vi "Test VI.vi"(9 "y":dbl, 10 "x":dbl) -> (0 "Application:Version Year":string, 1 "Application:Version Number":string, 2 "Application:Name":string, 3 "x+y":dbl)   [LabVIEW 2019]
uses:
  2018.lvlibp
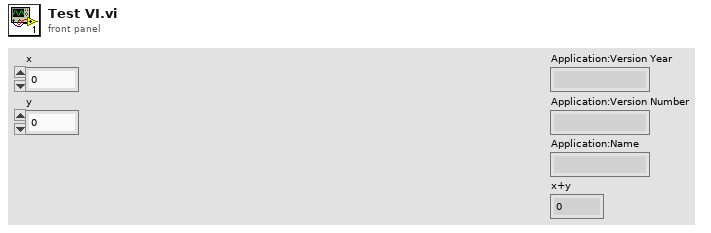
[diagram p1: front panel]
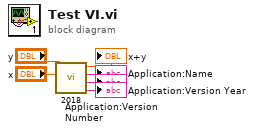
[diagram p0: block diagram]
diagram:
  n1 = call "2018.vi"("x"="x", "y"="y") -> ("Application:Version Year"=→"Application:Version Year":string, "Application:Version Number"=→"Application:Version Number":string, "Application:Name"=→"Application:Name":string, "x+y"=→"x+y":dbl)  [unwired: 6 in]
